vi "CheckListener ConvBox Handler.vi"(8 "error in (no error)":errorcluster, 11 "Listener in":refnum<class "Listener.lvclass">) -> (0 "error out":errorcluster, 3 "Listener out":refnum<class "Listener.lvclass">)   [LabVIEW 2019, in "Listener.lvclass"]
uses:
  Listener.lvclass
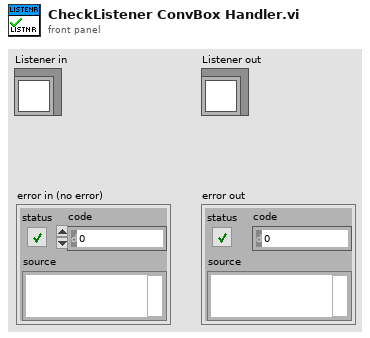
[diagram p1: front panel]
types:
  T1 = typedef "Listener.lvclass/RS-xxx To GPIB ConvBox Data Structure.ctl" = cluster{"Protocol Port Ref":refnum<visa-resource-name>, "Listener Port Ref":refnum<visa-resource-name>, "Data":string, "Command Messages Read":string[], "Address":string}
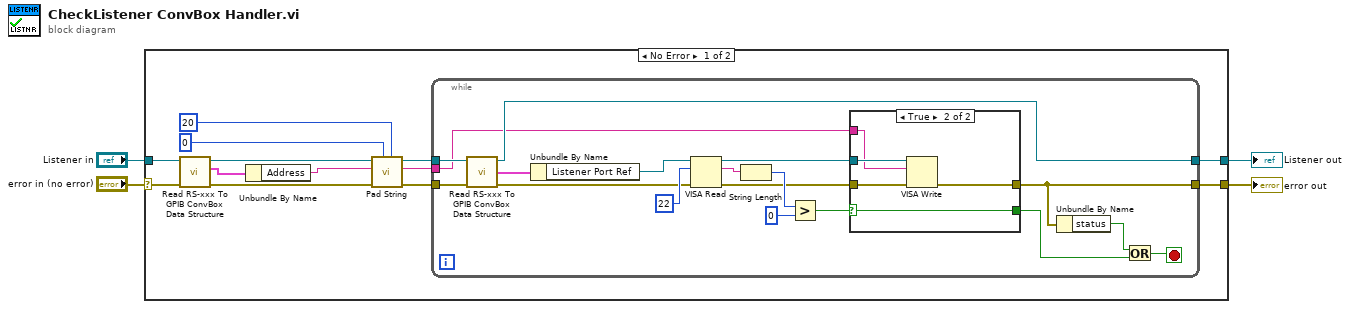
[diagram p0: block diagram]
diagram:
  n1 = case shown="No Error" "error in (no error)" {
    selector: "error in (no error)" -> [w14 w44]
    tunnel: [w17 w44] -> w4
    tunnel: "Listener in" -> [w15 w43]
    tunnel: [w16 w43] -> w1
    frame No Error {
      n2 = call-dynamic "Read RS-xxx To GPIB ConvBox Data Structure.vi"("error in (no error)"=w14, "Listener in"=w15) -> ("error out"=w12:errorcluster, "RS-xxx To GPIB ConvBox Data Structure"=w13:T1, "Listener out"=w9:refnum<class "Listener.lvclass">)  [unwired: 7 in]
      n3 = Unbundle By Name(w13) -> ("Address"=w10:string)
      n4 = call "Pad String.vi"("Expected Length"=u8 20, "Pad Character"=u8 0, "error in (no error)"=w12, "String To Pad"=w10, "Listener in"=w9) -> ("error out"=w11:errorcluster, "Padded String"=w6:string, "Listener out"=w5:refnum<class "Listener.lvclass">)  [unwired: 4 in]
      n5 = while {
        tunnel: w6 -> [w18]
        tunnel: w11 -> [w24]
        tunnel: [w29] -> w17
        tunnel: w5 -> [w23]
        tunnel: [w19] -> w16
        stop <- w28 stop-if-true
        n6 = call-dynamic "Read RS-xxx To GPIB ConvBox Data Structure.vi"("error in (no error)"=w24, "Listener in"=w23) -> ("error out"=w22:errorcluster, "RS-xxx To GPIB ConvBox Data Structure"=w21:T1, "Listener out"=w19:refnum<class "Listener.lvclass">)  [unwired: 7 in]
        n7 = Unbundle By Name(w21) -> ("Listener Port Ref"=w20:refnum<visa-resource-name>)
        n8 = VISA Read(VISA resource name=w20, byte count=u32 22, error in (no error)=w22) -> (VISA resource name out=w34:refnum<visa-resource-name>, read buffer=w33:string, error out=w25:errorcluster)  [unwired: 1 out]
        n9 = String Length(string=w33) -> (length=w32:i32)
        n10 = Greater?(x=w32, y=0) -> (0:w30:bool)
        n11 = case shown="True" w30 {
          selector: w30 -> [w37 w40]
          tunnel: w25 -> [w36 w42]
          tunnel: w34 -> [_ w41]
          tunnel: [w37 w40] -> w27
          tunnel: [w36 w39] -> w29
          tunnel: w18 -> [_ w38]
          frame False {
          }
          frame True {
            n12 = VISA Write(VISA resource name=w41, write buffer=w38, error in (no error)=w42) -> (error out=w39:errorcluster)  [unwired: 2 out]
          }
        }
        n13 = Unbundle By Name(w29) -> ("status"=w26:bool)
        n14 = Or(x=w26, y=w27) -> (x .or. y?=w28:bool)
      }
    }
    frame Error {
    }
  }
  "error out" <- w4
  "Listener out" <- w1
